vi "DAC Init Results.vi"(8 "error in":errorcluster, 9 "Log Details?":bool, 10 "tdms file":refnum<k34>, 11 "DAC TEG Temp in":refnum<class "DAC TEG Temp.lvclass">) -> (0 "error out":errorcluster, 2 "tdms file out":refnum<k34>)   [LabVIEW 2019, in "DAC.lvlib" / "DAC TEG Temp.lvclass"]
uses:
  DAC TEG Temp.lvclass
  C:/Users/wg/Documents/LV_Projects/test-stand/App/DAC/DAC.lvclass
  DAC.lvclass/DAC.ctl
  DAC TEG Temp.lvclass/DAC TEG Temp.ctl
  DAC.lvclass
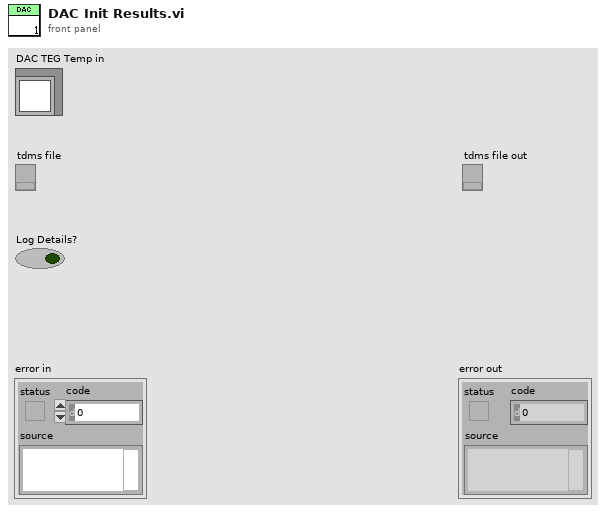
[diagram p1: front panel]
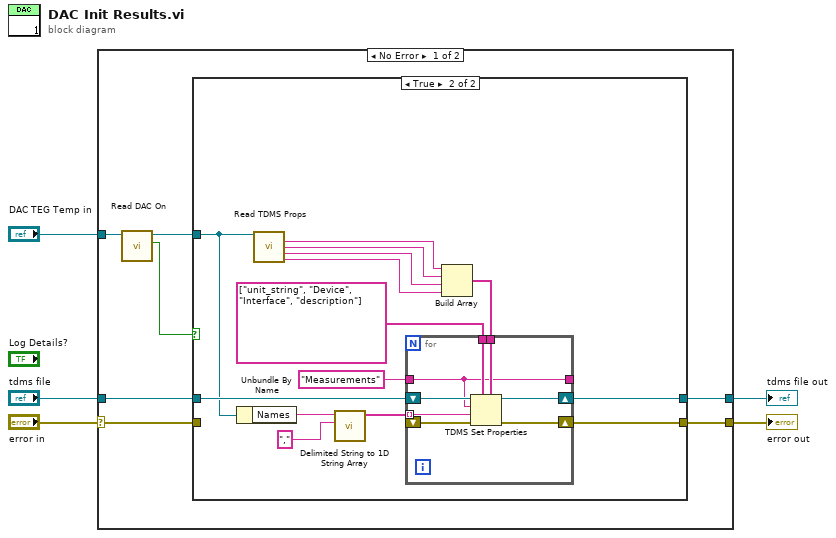
[diagram p0: block diagram]
diagram:
  n1 = case shown="No Error" "error in" {
    selector: "error in" -> [w9 w38]
    tunnel: [w6 w38] -> w2
    tunnel: "DAC TEG Temp in" -> [w12 _]
    tunnel: "tdms file" -> [w10 w37]
    tunnel: [w7 w37] -> w1
    frame No Error {
      n2 = call "Read DAC On.vi"("DAC in"=w12) -> ("DAC On"=w11:bool, "DAC out"=w8:refnum<class "DAC TEG Temp.lvclass">)  [unwired: 8 in, 1 out]
      n3 = case shown="True" w11 {
        tunnel: w10 -> [w14 w28]
        tunnel: [w14 w16] -> w7
        tunnel: [w13 w15] -> w6
        tunnel: w8 -> [_ w19]
        tunnel: w9 -> [w13 _]
        frame False {
        }
        frame True {
          n4 = Unbundle By Name(w19) -> ("Names"=w25:string)
          n5 = call "Read TDMS Props.vi"("DAC in"=w19) -> ("Result Unit"=w24:string, "DAC Device"=w23:string, "DAC IO"=w22:string, "DAC Description"=w21:string)  [unwired: 10 in, 1 out]
          n6 = call <vilib>:"Delimited String to 1D String Array.vi"("delimiter"=",", "delimited string"=w25) -> ("string array"=w27:string[])  [unwired: 9 in]
          n7 = Build Array(w24, w23, w22, w21) -> (w18:string[])
          n8 = for {
            tunnel: w27 -> [w31] mode=indexing
            tunnel: string[] ["unit_string", "Device", "Interface", "description"] ("property names") -> [w33]
            tunnel: w18 -> [w32]
            shift-right: [w34] -> w16
            shift-left: w28 -> [w36]
            tunnel: "Measurements" ("group name in (Untitled)") -> [w29]
            shift-right: [w35] -> w15
            shift-left: _ -> [w30]
            tunnel: [w29] -> _
            n9 = TDMS Set Properties(5:w32, 7:w33, 8:w30, 9:w31, 10:w29, 11:w36) -> (0:w35:errorcluster, 3:w34:refnum<k34>)  [unwired: 2 out]
          }
        }
      }
    }
    frame Error {
    }
  }
  "error out" <- w2
  "tdms file out" <- w1
